vi "WIP.vi"() -> ()   [LabVIEW 2020]
uses:
  <vilib>/userdefined/High Color/IMAQdx.ctl
  Supporting Files/Sensor Station States.ctl
  Keyence CL-3000/Public/clusters/CL3IF_MEASUREMENT_DATA.ctl
  Keyence CL-3000/Public/clusters/CL3IF_OUTMEASUREMENT_DATA.ctl
  Keyence CL-3000/Public/enums/CL3IF_VALUE_INFO.ctl
  Keyence CL-3000/Public/enums/CL3IF_JUDGE_RESULT.ctl
  Keyence CL-3000/Public/clusters/CL3IF_ETHERNET_SETTING.ctl
  Keyence CL-3000/Keyence CL-3000.lvlib
  <vilib>/WebDAVClient/NI_WebDAV.lvlib
  <vilib>/vision/driver/NI_Vision_Acquisition_Software.lvlib
  <vilib>/WebDAVClient/Advanced/Multi Event/Asynchronous Get File.vi
panel:
  in  "Select Camera":T1
  in  "Enable Camera":bool
  in  "Visualise \nLaser":bool
  out "Numeric":i32
  out "Confocal\nSave Error":errorcluster
  in  "Visualise\nChromatic":bool
  in  "Log Laser Data":bool
  out "Laser Displacement Readings (cRIO) 2":dbl(graph)
  in  "Enable Laser":bool
  in  "Filename":string
  in  "Save Location (Folder)":path
  out "Chromatic Logged Data Points":u32
  in  "IP Address":u8[](array[numeric])=[192, 168, 1, 1]
  in  "Port":u32
  in  "timeout":u32=5000 caption="Timeout"
  in  "Comm Interface":enum8{"USB", "ETHERNET"}(ring)
  in  "Device ID":i32 min=0 max=2
  out "Confocal Data Index 2":u32
  in  "Log Chromatic Data":bool
  in  "Enable Chromatic":bool
  out "Confocal Data Index 1":u32
  in  "STOP":bool
  out "Camera Feed":T2(plugin-control)
  in  "Capture Image":bool
  out "Captured Image":T2(plugin-control)
  out "Measurement Data":T3(array[cluster])=[{"Out No"=1, "Value"=0, "valueInfo"=enum."VALID", "judgeResult"=0}, {"Out No"=2, "Value"=0, "valueInfo"=enum."VALID", "judgeResult"=0}, {"Out No"=3, "Value"=0, "valueInfo"=enum."VALID", "judgeResult"=0}, {"Out No"=4, "Value"=0, "valueInfo"=enum."VALID", "judgeResult"=0}, {"Out No"=5, "Value"=0, "valueInfo"=enum."VALID", "judgeResult"=0}, {"Out No"=6, "Value"=0, "valueInfo"=enum."VALID", "judgeResult"=0}, {"Out No"=7, "Value"=0, "valueInfo"=enum."VALID", "judgeResult"=0}, {"Out No"=8, "Value"=0, "valueInfo"=enum."VALID", "judgeResult"=0}] {"judgeResult" items=["HI"=1, "GO"=2, "LO"=4, "**"=5, "--"=0]}
  out "Chromatic Confocal Readings":dbl(graph)
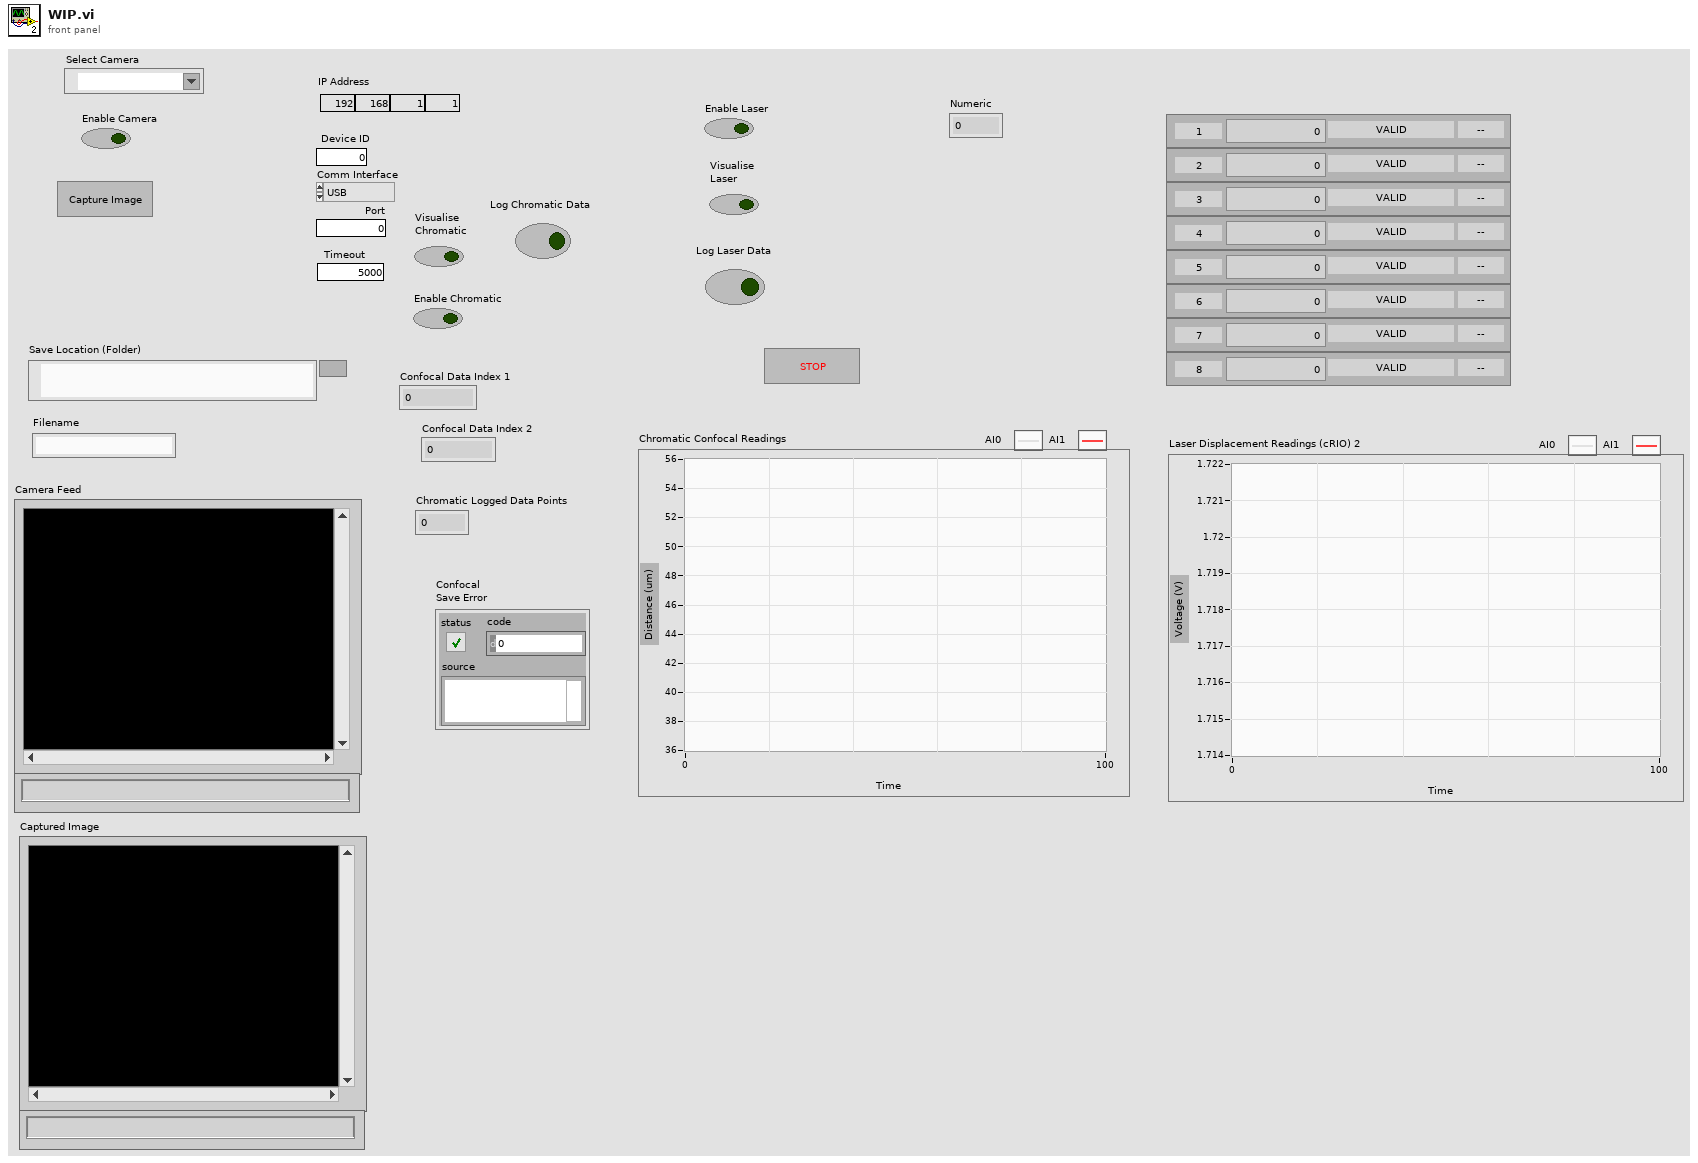
[diagram p1: front panel]
types:
  T1 = typedef "IMAQdx.ctl" = refnum<k21>
  T2 = typedef "IMAQ Image.ctl" = refnum<image>
  T3 = cluster{"Out No":i32, "Value":i32, "valueInfo":enum8{"VALID", "JUDGMENTSTANDBY", "INVALID", "OVERDISPRANGE_P", "OVERDISPRANGE_N"}, "judgeResult":u16}[]
  T4 = typedef "Keyence CL-3000.lvlib/CL3IF_MEASUREMENT_DATA.ctl" = cluster{"addInfo":cluster{"triggerCount":u32, "pulseCount":i32}, "outMeasurementData":T5[]}
  T5 = typedef "Keyence CL-3000.lvlib/CL3IF_OUTMEASUREMENT_DATA.ctl" = cluster{"measurementValue":i32, "valueInfo":T6, "judgeResult":T7}
  T6 = typedef "Keyence CL-3000.lvlib/CL3IF_VALUE_INFO.ctl" = enum8{"VALID", "JUDGMENTSTANDBY", "INVALID", "OVERDISPRANGE_P", "OVERDISPRANGE_N"}
  T7 = typedef "Keyence CL-3000.lvlib/CL3IF_JUDGE_RESULT.ctl" = u8
  T8 = typedef "Sensor Station States.ctl" = enum16{"Initialise", "Acquire", "Visualise", "Log", "Save", "Check Time", "Idle", "Close"}
  T9 = enum16{"open", "replace", "create", "open or create", "replace or create", "replace or create with confirmation"}
  T10 = typedef "NI_WebDAV.lvlib/Asynchronous Session Handle.ctl" = refnum<k1>
  T11 = typedef "Keyence CL-3000.lvlib/CL3IF_ETHERNET_SETTING.ctl" = cluster{"IP Address":cluster{"IP1":u8, "IP2":u8, "IP3":u8, "IP4":u8}, "portNo":u32}
  T12 = cluster{"IP Address":u8, "IP Address":u8, "IP Address":u8, "IP Address":u8}
  T13 = cluster{i32, "measurementValue":i32, "valueInfo":T6, "judgeResult":T7}
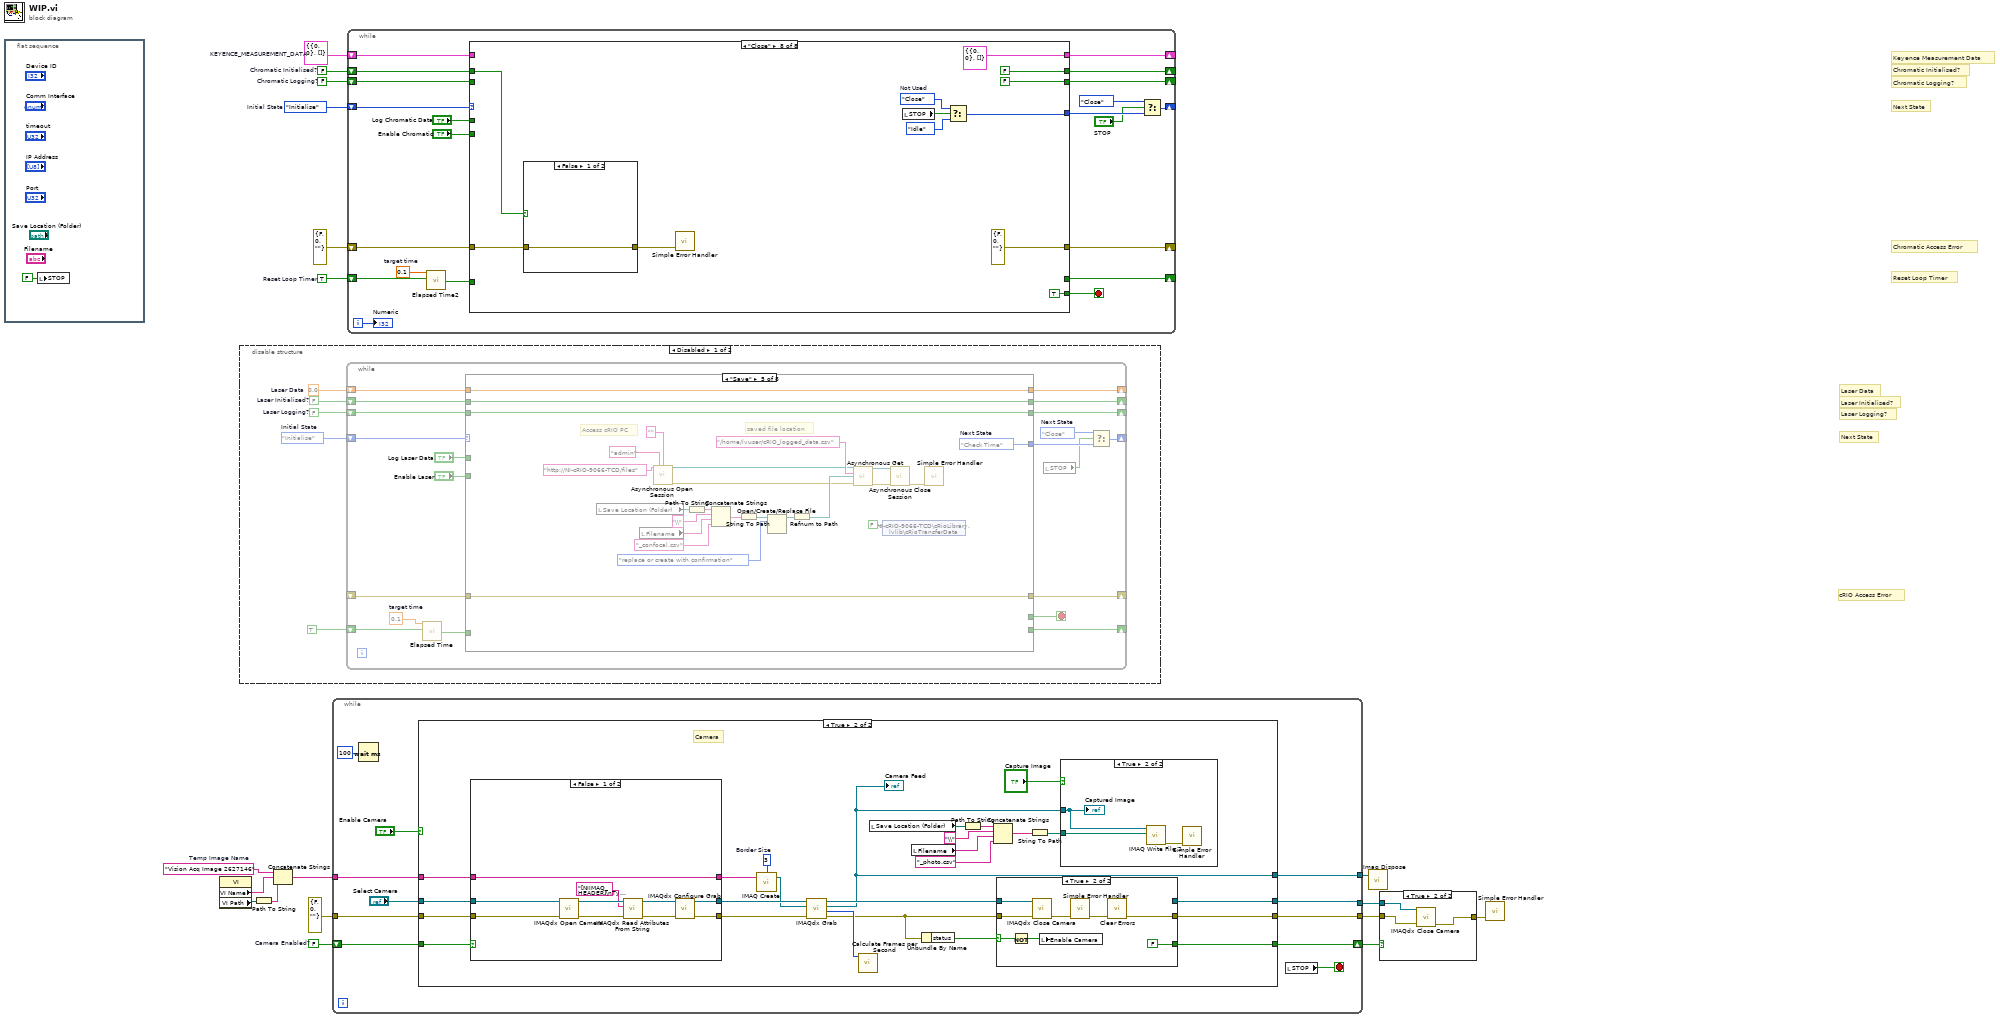
[diagram p0: block diagram]
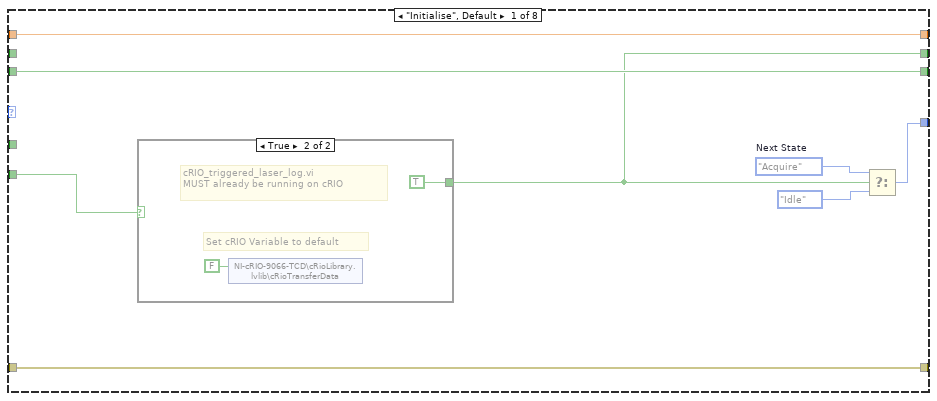
[diagram p3: hidden frame]
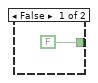
[diagram p4: hidden frame]
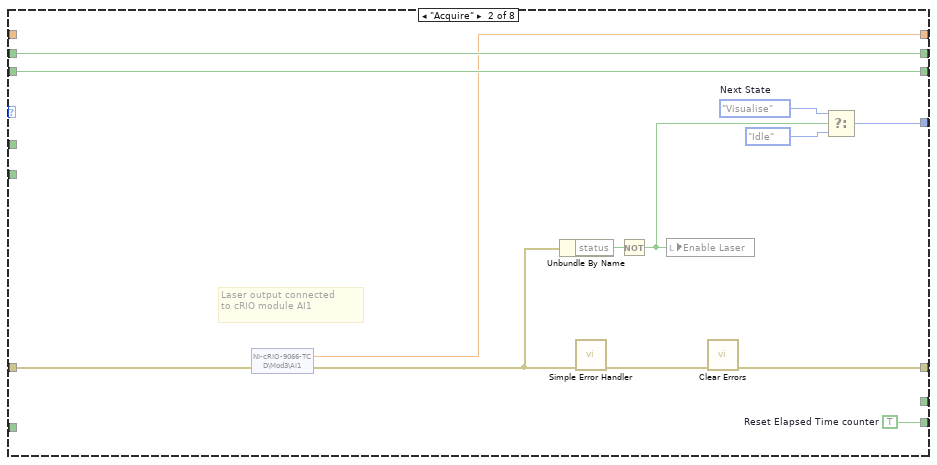
[diagram p5: hidden frame]
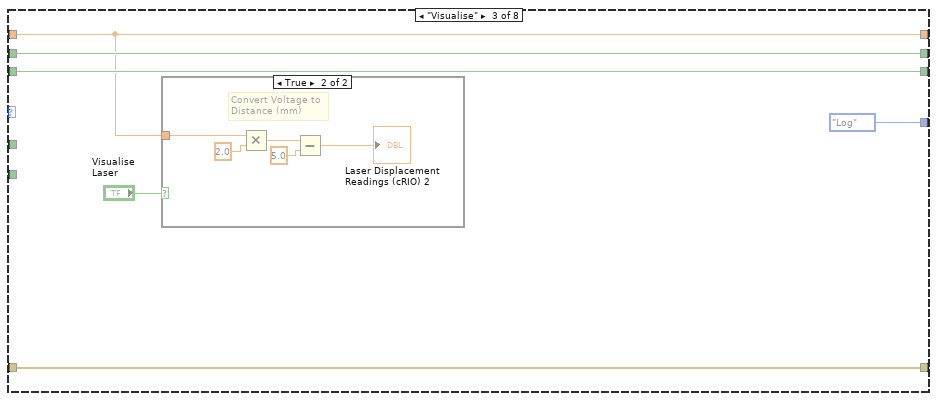
[diagram p6: hidden frame]
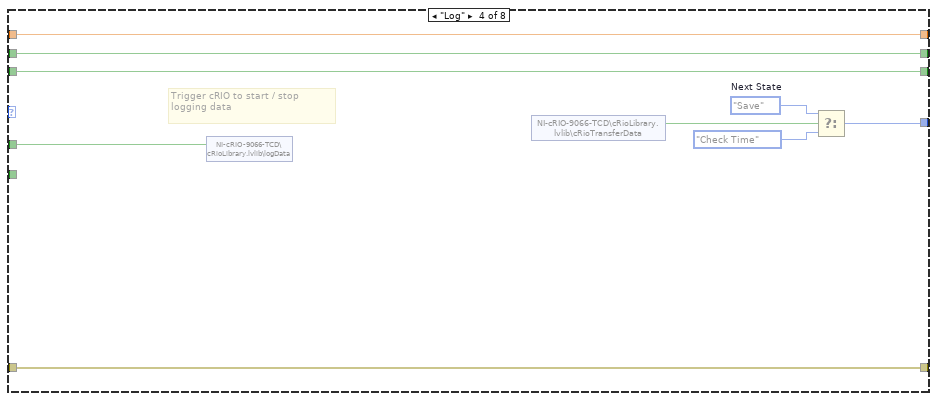
[diagram p8: hidden frame]
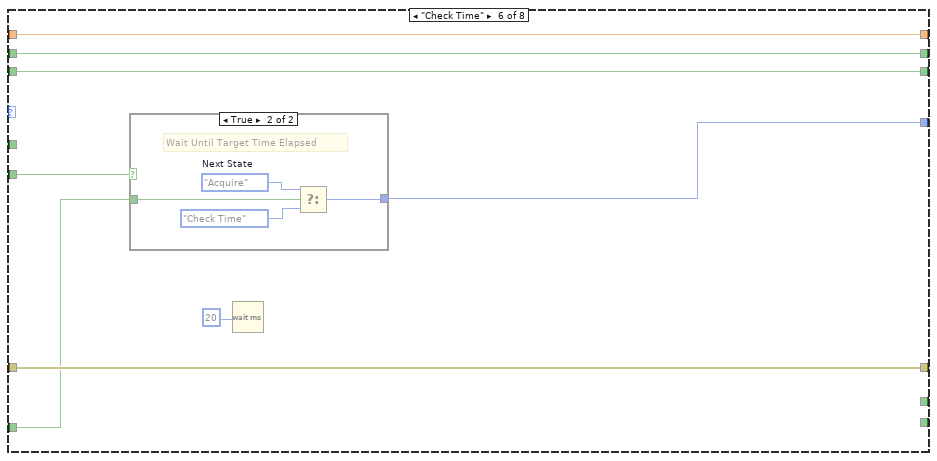
[diagram p9: hidden frame]
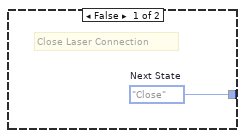
[diagram p10: hidden frame]
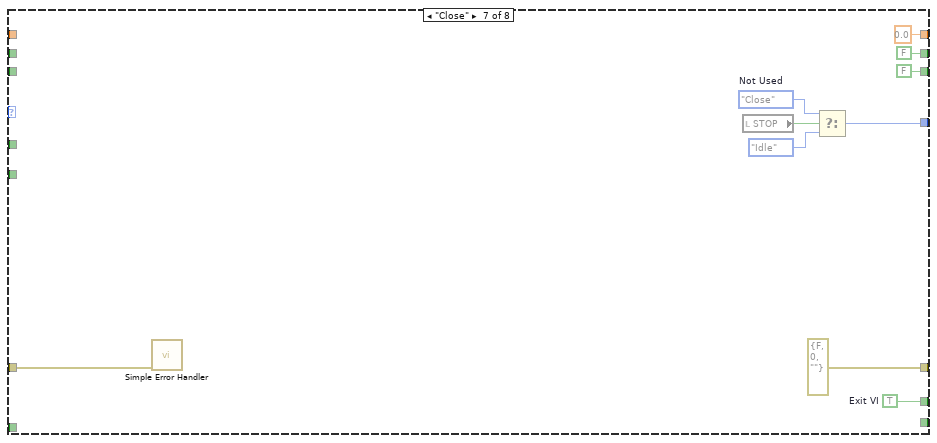
[diagram p11: hidden frame]
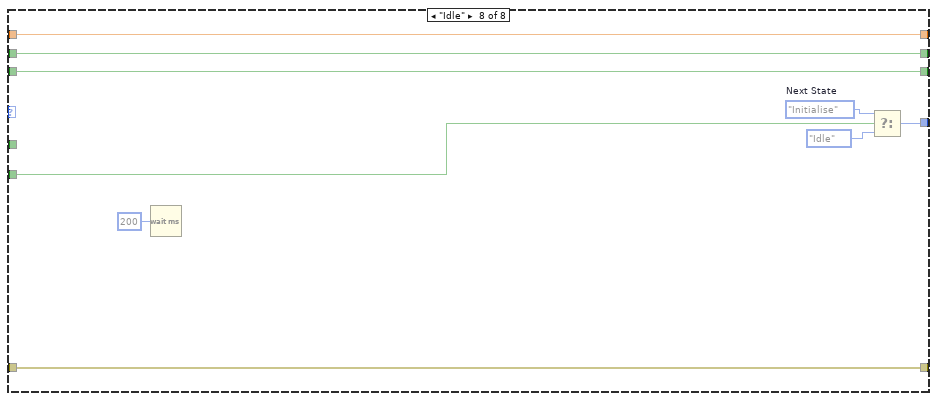
[diagram p12: hidden frame]
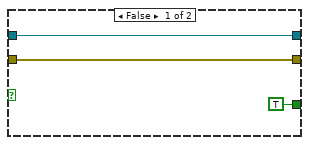
[diagram p16: hidden frame]
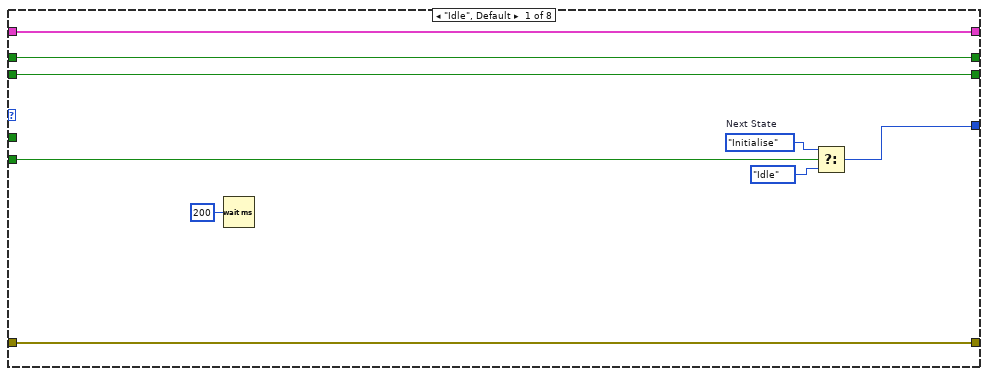
[diagram p18: hidden frame]
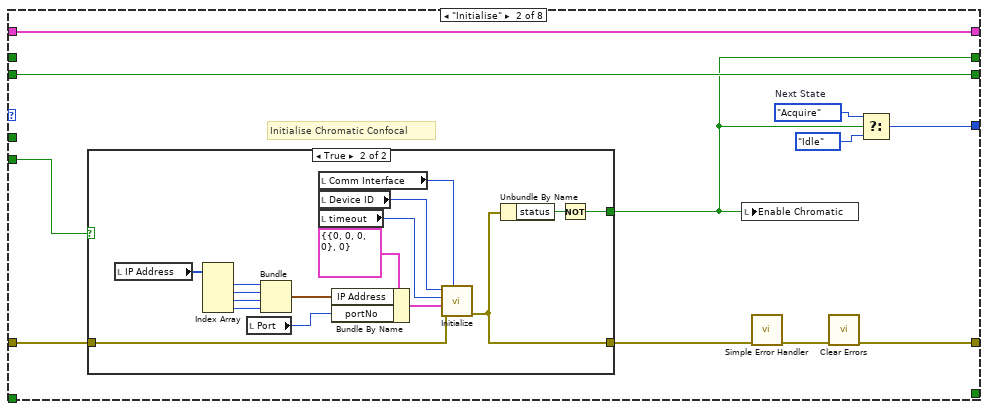
[diagram p19: hidden frame]
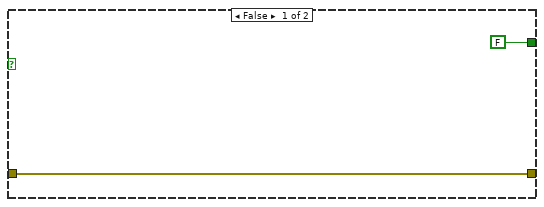
[diagram p20: hidden frame]
diagram:
  w7 = "Vision Acq Image 2627146"  # Temp Image Name
  w11 = FALSE  # Camera Enabled?
  w14 = FALSE  # Chromatic Initialised?
  w15 = FALSE  # Chromatic Logging?
  w16 = TRUE  # Reset Loop Timer
  w17 = T4 {"addInfo"={"triggerCount"=0, "pulseCount"=0}, "outMeasurementData"=[]}  # KEYENCE_MEASUREMENT_DATA
  w18 = Sensor_Station_States."Initialise"  # Initial State
  # "cRIO Access Error"
  # "Next State"
  # "Laser Logging?"
  # "Laser Initialised?"
  # "Laser Data"
  # "Reset Loop Timer"
  # "Chromatic Access Error"
  # "Next State"
  # "Keyence Measurement Data"
  # "Chromatic Logging?"
  # "Chromatic Initialised?"
  n1 = flat-sequence {
    frame #0 {
      n2 = local write "STOP"(FALSE ("STOP")) -> ()
    }
  }
  n3 = property class="VI"() -> ("VI Name"=w9:string, "VI Path"=w8:path)  [unwired: 2 in, 2 out]
  n4 = disable-structure shown="Disabled" {
    frame Disabled {
      w20 = 0.0  # Laser Data
      w21 = FALSE  # Laser Initialised?
      w24 = FALSE  # Laser Logging?
      w22 = Sensor_Station_States."Initialise"  # Initial State
      n5 = while {
        shift-right: [w31] -> _
        shift-left: w22 -> [w44]
        shift-right: [w40] -> _
        shift-left: TRUE -> [w42]
        shift-right: [w38] -> _
        shift-left: w24 -> [w39]
        shift-right: [w37] -> _
        shift-left: _ -> [w36]
        shift-right: [w35] -> _
        shift-left: w21 -> [w34]
        shift-right: [w27] -> _
        shift-left: w20 -> [w26]
        stop <- w30 stop-if-true
        w32 = Sensor_Station_States."Close"  # Next State
        w43 = 0.1  # target time
        n6 = call "Elapsed Time"("Time Target (s)"=w43, "Reset"=w42) -> ("Time has Elapsed"=w41:bool)  [unwired: 10 in, 7 out]
        n7 = case shown="\"Save\"" w44 {
          tunnel: w36 -> [w46 w67 w73 w83 w113 w118 w127 w140]
          tunnel: [w51 w57 Sensor_Station_States."Log" ("Next State") w86 w112 w115 w129 w142] -> w33
          tunnel: w41 -> [_ _ _ _ _ w116 _ _]
          tunnel: [_ w68 _ _ _ _ _ _] -> w40
          tunnel: w39 -> [w50 w65 w72 w81 w109 w120 _ w138]
          tunnel: [w50 w65 w72 w81 w109 w120 FALSE ("Chromatic Logging?") w138] -> w38
          tunnel: [w46 w62 w73 w83 w113 w118 errorcluster {"status"=FALSE, "code"=0, "source"=""} ("error constant") w140] -> w37
          tunnel: [w48 w66 w74 w88 w110 w119 FALSE w139] -> w35
          tunnel: w34 -> [_ w66 w74 w88 w110 w119 _ w139]
          tunnel: [_ _ _ _ _ _ w136 _] -> w30
          tunnel: "Enable Laser" -> [w49 _ _ _ _ w117 _ w143]
          tunnel: [w45 w64 w69 w82 w111 w114 0.0 w137] -> w27
          tunnel: w26 -> [w45 _ w69 w82 w111 w114 _ w137]
          tunnel: "Log Laser Data" -> [_ _ _ w84 _ _ _ _]
          frame "Initialise", Default {
            w47 = Sensor_Station_States."Acquire"  # Next State
            n8 = case shown="True" w49 {
              tunnel: [FALSE TRUE] -> w48
              frame False {
              }
              frame True {
                # "cRIO_triggered_laser_log.vi \nMUST already be running on cRIO"
                # "Set cRIO Variable to default"
                n9 = shared-variable "NI-cRIO-9066-TCD\\cRioLibrary.lvlib\\cRioTransferData"(FALSE ("cRioTransferData")) -> ()  [unwired: 1 in, 1 out]
              }
            }
            n10 = Select(t=w47, s=w48, f=Sensor_Station_States."Idle" ("Next State")) -> (s? t:f=w51:T8)
          }
          frame "Acquire" {
            w68 = TRUE  # Reset Elapsed Time counter
            w58 = Sensor_Station_States."Visualise"  # Next State
            # "Laser output connected \nto cRIO module AI1"
            n11 = shared-variable "NI-cRIO-9066-TCD\\Mod3\\AI1"(error in=w67) -> (w64:dbl, error out=w60:errorcluster)
            n12 = Unbundle By Name(w60) -> ("status"=w61:bool)
            n13 = call <vilib>:"Simple Error Handler.vi"("error in (no error)"=w60) -> ("error out"=w63:errorcluster)  [unwired: 4 in, 4 out]
            n14 = Not(x=w61) -> (.not. x?=w59:bool)
            n15 = local write "Enable Laser"(w59) -> ()
            n16 = call <vilib>:"Clear Errors.vi"("error in (no error)"=w63) -> ("error out"=w62:errorcluster)  [unwired: 5 in, 1 out]
            n17 = Select(t=w58, s=w59, f=Sensor_Station_States."Idle" ("Next State")) -> (s? t:f=w57:T8)
          }
          frame "Visualise" {
            n18 = case shown="True" "Visualise \nLaser" {
              tunnel: w69 -> [_ w75]
              frame False {
                # "Do nothing"
              }
              frame True {
                # "Convert Voltage to Distance (mm)"
                n19 = Multiply(x=w75, y=2.0) -> (x*y=w78:dbl)
                n20 = Subtract(x=w78, y=5.0) -> (x-y=→"Laser Displacement Readings (cRIO) 2":dbl)
              }
            }
          }
          frame "Log" {
            w87 = Sensor_Station_States."Save"  # Next State
            # "Trigger cRIO to start / stop \nlogging data"
            n21 = shared-variable "NI-cRIO-9066-TCD\\cRioLibrary.lvlib\\logData"(w84) -> ()  [unwired: 1 in, 1 out]
            n22 = shared-variable "NI-cRIO-9066-TCD\\cRioLibrary.lvlib\\cRioTransferData"() -> (w80:bool)  [unwired: 1 in, 1 out]
            n23 = Select(t=w87, s=w80, f=Sensor_Station_States."Check Time" ("Next State")) -> (s? t:f=w86:T8)
          }
          frame "Save" {
            w112 = Sensor_Station_States."Check Time"  # Next State
            # "Access cRIO PC"
            # "saved file location"
            n24 = local read "Save Location (Folder)"() -> (w106:path)
            n25 = local read "Filename"() -> (w103:string)
            n26 = call <vilib>:"Asynchronous Open Session.vi"("host uri prefix"="http://NI-cRIO-9066-TCD/files", "username"="admin", "password"="") -> ("session handle out"=w93:T10, "error out"=w92:errorcluster)  [unwired: 10 in, 1 out]
            n27 = Path To String(path=w106) -> (string=w105:string)
            n28 = Concatenate Strings(w105, "\\" ("string"), w103, "_confocal.csv" ("string")) -> (w101:string)
            n29 = String To Path(string=w101) -> (path=w100:path)
            n30 = Open/Create/Replace File(file path (use dialog)=w100, operation (0:open)=T9."replace or create with confirmation") -> (refnum out=w98:refnum<file>)  [unwired: 4 in, 2 out]
            n31 = Refnum to Path(1:w98) -> (0:w97:path)
            n32 = call-poly <vilib>:"Asynchronous Get.vi"("session handle"=w93, "relative uri"="/home/lvuser/cRIO_logged_data.csv", "local file path"=w97, "error in (no error)"=w92) -> ("session handle out"=w90:T10, "error out"=w89:errorcluster)  [unwired: 8 in, 2 out]
            n33 = shared-variable "NI-cRIO-9066-TCD\\cRioLibrary.lvlib\\cRioTransferData"(FALSE ("cRioTransferData")) -> ()  [unwired: 1 in, 1 out]
            n34 = call <vilib>:"Asynchronous Close Session.vi"("session handle"=w90, "error in (no error)"=w89) -> ("error out"=w91:errorcluster)  [unwired: 13 in]
            n35 = call <vilib>:"Simple Error Handler.vi"("error in (no error)"=w91) -> ()  [unwired: 4 in, 5 out]
          }
          frame "Check Time" {
            n36 = case shown="True" w117 {
              tunnel: w116 -> [_ w124]
              tunnel: [w122 w123] -> w115
              frame False {
                w122 = Sensor_Station_States."Close"  # Next State
                # "Close Laser Connection"
              }
              frame True {
                w125 = Sensor_Station_States."Acquire"  # Next State
                # "Wait Until Target Time Elapsed"
                n37 = Select(t=w125, s=w124, f=Sensor_Station_States."Check Time" ("Next State")) -> (s? t:f=w123:T8)
              }
            }
            n38 = Wait (ms)(milliseconds to wait=u32 20) -> ()  [unwired: 1 out]
          }
          frame "Close" {
            w131 = Sensor_Station_States."Close"  # Not Used
            w136 = TRUE  # Exit VI
            n39 = call <vilib>:"Simple Error Handler.vi"("error in (no error)"=w127) -> ()  [unwired: 4 in, 5 out]
            n40 = local read "STOP"() -> (w130:bool)
            n41 = Select(t=w131, s=w130, f=Sensor_Station_States."Idle" ("Next State")) -> (s? t:f=w129:T8)
          }
          frame "Idle" {
            w145 = Sensor_Station_States."Initialise"  # Next State
            n42 = Wait (ms)(milliseconds to wait=u32 200) -> ()  [unwired: 1 out]
            n43 = Select(t=w145, s=w143, f=Sensor_Station_States."Idle" ("Next State")) -> (s? t:f=w142:T8)
          }
        }
        n44 = local read "STOP"() -> (w29:bool)
        n45 = Select(t=w32, s=w29, f=w33) -> (s? t:f=w31:T8)
      }
    }
    frame Enabled {
    }
  }
  n46 = Path To String(path=w8) -> (string=w10:string)
  n47 = Concatenate Strings(w7, w9, w10) -> (w6:string)
  n48 = while {
    tunnel: [w156] -> w12
    tunnel: [w155] -> w3
    shift-right: [w147] -> w1
    shift-left: w11 -> [w151]
    tunnel: errorcluster {"status"=FALSE, "code"=0, "source"=""} ("error in") -> [w149]
    tunnel: w6 -> [w150]
    tunnel: [w146] -> w4
    stop <- w152 stop-if-true
    n49 = Wait (ms)(milliseconds to wait=u32 100) -> ()  [unwired: 1 out]
    n50 = case shown="True" "Enable Camera" {
      tunnel: [w158 w183] -> w155
      tunnel: [_ w170] -> w156
      tunnel: w151 -> [w157 w169]
      tunnel: w150 -> [_ w164]
      tunnel: w149 -> [w158 w168]
      tunnel: "Select Camera" -> [w159 w163]
      tunnel: [w157 w161] -> w147
      tunnel: [w159 w160] -> w146
      frame False {
      }
      frame True {
        w167 = 3  # Border Size
        # "Camera"
        n51 = case shown="False" w169 {
          tunnel: [w194 w196] -> w177
          tunnel: [w193 w195] -> w176
          tunnel: w168 -> [w187 w195]
          tunnel: [w186 w197] -> w165
          tunnel: w164 -> [w186 w197]
          tunnel: w163 -> [w185 w196]
          frame False {
            n52 = call <vilib>:"IMAQdx Open Camera.vi"("error in"=w187, "Session In"=w185) -> ("error out"=w191:errorcluster, "Session Out"=w192:T1)  [unwired: 1 in, 7 out]
            n53 = call <vilib>:"IMAQdx Read Attributes From String.vi"("error in"=w191, "Attributes String In"="[NIIMAQ_HEADER]\nType = 2\nVersion = 8\n\n[CAMERA_DATA]\nAcquisitionAttributes::Bayer::Algorithm = \"Bilinear\"\nAcquisitionAttributes::Bayer::GainB = \"1\"\nAcquisitionAttributes::Bayer::GainG = \"1\"\nAcquisitionAttributes::Bayer::GainR = \"1\"\nAcquisitionAttributes::Bayer::Pattern = \"Use hardware value\"\nAcquisitionAttributes::BitsPerPixel = \"Use hardware value\"\nAcquisitionAttributes::HardwareMaximumQueuedBufferCount = \"1000\"\nAcquisitionAttributes::HardwareRequeueBufferListThreshold = \"50\"\nAcquisitionAttributes::IgnoreFirstFrame = \"false\"\nAcquisitionAttributes::ImageDecoderCopyMode = \"Auto\"\nAcquisitionAttributes::OutputImageType = \"Auto\"\nAcquisitionAttributes::OverwriteMode = \"Get Newest\"\nAcquisitionAttributes::PixelSignedness = \"Use hardware value\"\nAcquisitionAttributes::ReceiveTimestampMode = \"None\"\nAcquisitionAttributes::ShiftPixelBits = \"false\"\nAcquisitionAttributes::SwapPixelBytes = \"false\"\nAcquisitionAttributes::Timeout = \"5000\"\nAcquisitionAttributes::VerticalMirror = \"false\"\nAcquisitionAttributes::VideoMode = \"640x480 YUY2 30.00fps\"\nCameraAttributes::BacklightCompensation::Mode = \"Manual\"\nCameraAttributes::BacklightCompensation::Value = \"true\"\nCameraAttributes::Brightness::Mode = \"Manual\"\nCameraAttributes::Brightness::Value = \"0\"\nCameraAttributes::Contrast::Mode = \"Manual\"\nCameraAttributes::Contrast::Value = \"0.179999999999999993\"\nCameraAttributes::Exposure::Mode = \"Auto\"\nCameraAttributes::Gain::Mode = \"Manual\"\nCameraAttributes::Gain::Value = \"1\"\nCameraAttributes::Gamma::Mode = \"Manual\"\nCameraAttributes::Gamma::Value = \"1.5\"\nCameraAttributes::Hue::Mode = \"Manual\"\nCameraAttributes::Hue::Value = \"0\"\nCameraAttributes::Saturation::Mode = \"Manual\"\nCameraAttributes::Saturation::Value = \"8\"\nCameraAttributes::Sharpness::Mode = \"Manual\"\nCameraAttributes::Sharpness::Value = \"3\"\nCameraAttributes::WhiteBalance::Mode = \"Auto\"\n" ("Attributes"), "Session In"=w192) -> ("error out"=w189:errorcluster, "Session Out"=w190:T1)  [unwired: 7 out]
            n54 = call <vilib>:"IMAQdx Configure Grab.vi"("error in"=w189, "Session In"=w190) -> ("error out"=w193:errorcluster, "Session Out"=w194:T1)  [unwired: 1 in, 7 out]
          }
          frame True {
            # "Camera Initialised"
          }
        }
        n55 = call "IMAQ Create"("Border Size"=w167, "Image Name"=w165) -> ("New Image"=w166:T2)  [unwired: 2 in, 2 out]
        n56 = call <vilib>:"IMAQdx Grab.vi"("error in"=w176, "Image In"=w166, "Session In"=w177) -> ("error out"=w178:errorcluster, "Buffer Number Out"=w179:u32, "Image Out"=w170:T2, "Session Out"=w180:T1)  [unwired: 1 in, 4 out]
        "Camera Feed" <- w170
        n57 = call <vilib>:"Calculate Frames per Second.vi"("Buffer Number"=w179) -> ()  [unwired: 2 in, 9 out]
        n58 = local read "Save Location (Folder)"() -> (w175:path)
        n59 = local read "Filename"() -> (w172:string)
        n60 = Unbundle By Name(w178) -> ("status"=w162:bool)
        n61 = Path To String(path=w175) -> (string=w174:string)
        n62 = Concatenate Strings(w174, "\\" ("string"), w172, "_photo.csv" ("string")) -> (w182:string)
        n63 = case "Case Structure_template1" shown="True" w162 {
          selector: w162 -> [_ w203]
          tunnel: [w200 w204] -> w183
          tunnel: w178 -> [w200 w208]
          tunnel: w180 -> [w198 w206]
          tunnel: [TRUE FALSE] -> w161
          tunnel: [w198 _] -> w160
          frame False {
          }
          frame True {
            n64 = Not(x=w203) -> (.not. x?=w202:bool)
            n65 = call <vilib>:"IMAQdx Close Camera.vi"("error in"=w208, "Session In"=w206) -> ("error out"=w207:errorcluster)  [unwired: 9 out]
            n66 = local write "Enable Camera"(w202) -> ()
            n67 = call <vilib>:"Simple Error Handler.vi"("error in (no error)"=w207) -> ("error out"=w205:errorcluster)  [unwired: 4 in, 4 out]
            n68 = call <vilib>:"Clear Errors.vi"("error in (no error)"=w205) -> ("error out"=w204:errorcluster)  [unwired: 5 in, 1 out]
          }
        }
        n69 = String To Path(string=w182) -> (path=w181:path)
        n70 = case shown="True" "Capture Image" {
          tunnel: w170 -> [_ w211]
          tunnel: w181 -> [_ w210]
          frame False {
          }
          frame True {
            n71 = call-poly "IMAQ Write File 2"("File Path"=w210, "Image"=w211) -> ("error out"=w209:errorcluster)  [unwired: 8 in, 1 out]
            n72 = call <vilib>:"Simple Error Handler.vi"("error in (no error)"=w209) -> ()  [unwired: 4 in, 5 out]
            "Captured Image" <- w211
          }
        }
      }
    }
    n73 = local read "STOP"() -> (w152:bool)
  }
  n74 = while {
    shift-right: [w217] -> _
    shift-left: w18 -> [w232]
    shift-right: [w230] -> _
    shift-left: w17 -> [w231]
    shift-right: [w226] -> _
    shift-left: w16 -> [w228]
    shift-right: [w224] -> _
    shift-left: w15 -> [w225]
    shift-right: [w223] -> _
    shift-left: errorcluster {"status"=FALSE, "code"=0, "source"=""} ("error constant") -> [w222]
    shift-right: [w221] -> _
    shift-left: w14 -> [w220]
    i -> [w212]
    stop <- w216 stop-if-true
    w229 = 0.1  # target time
    n75 = call "Elapsed Time2"("Time Target (s)"=w229, "Reset"=w228) -> ("Time has Elapsed"=w227:bool)  [unwired: 10 in, 7 out]
    n76 = case shown="\"Close\"" w232 {
      tunnel: w231 -> [w240 w252 _ w279 w308 w352 w377 _]
      tunnel: w222 -> [w234 w248 w276 w283 w311 w342 w380 w400]
      tunnel: [w240 w252 w272 w279 w308 w352 w377 T4 {"addInfo"={"triggerCount"=0, "pulseCount"=0}, "outMeasurementData"=[]} ("KEYENCE_MEASUREMENT_DATA")] -> w230
      tunnel: [w237 w250 w275 Sensor_Station_States."Log" ("Next State") w304 w341 w378 w393] -> w219
      tunnel: w227 -> [_ _ _ _ _ _ w379 _]
      tunnel: [_ _ w278 _ _ _ _ _] -> w226
      tunnel: w225 -> [w233 w249 w277 w282 w312 w339 w382 _]
      tunnel: [w233 w249 w277 w282 w310 w339 w382 FALSE ("Chromatic Logging?")] -> w224
      tunnel: [w234 w244 w273 w283 w301 w342 w380 errorcluster {"status"=FALSE, "code"=0, "source"=""} ("error constant")] -> w223
      tunnel: [w241 w243 w271 w284 w309 w340 w381 FALSE] -> w221
      tunnel: w220 -> [w241 _ w271 w284 w309 w340 w381 w392]
      tunnel: [_ _ _ _ _ _ _ TRUE ("Exit VI")] -> w216
      tunnel: "Enable Chromatic" -> [w236 w246 _ _ _ _ w376 _]
      tunnel: "Log Chromatic Data" -> [_ _ _ _ w303 _ _ _]
      frame "Idle", Default {
        w239 = Sensor_Station_States."Initialise"  # Next State
        n77 = Wait (ms)(milliseconds to wait=u32 200) -> ()  [unwired: 1 out]
        n78 = Select(t=w239, s=w236, f=Sensor_Station_States."Idle" ("Next State")) -> (s? t:f=w237:T8)
      }
      frame "Initialise" {
        w251 = Sensor_Station_States."Acquire"  # Next State
        # "Initialise Chromatic Confocal"
        n79 = case shown="True" w246 {
          tunnel: [w253 w257] -> w245
          tunnel: [FALSE w256] -> w243
          tunnel: w248 -> [w253 w258]
          frame False {
          }
          frame True {
            n80 = local read "IP Address"() -> (w260:u8[])
            n81 = Index Array(array=w260) -> (element #1=w265:u8, element #2=w266:u8, element #3=w267:u8, element #4=w268:u8)  [unwired: 4 in]
            n82 = local read "Port"() -> (w259:u32)
            n83 = Bundle("IP Address"=w265, "IP Address"=w266, "IP Address"=w267, "IP Address"=w268) -> (w269:T12)  [unwired: 1 in]
            n84 = local read "Comm Interface"() -> (w262:enum8{"USB", "ETHERNET"})
            n85 = local read "Device ID"() -> (w263:i32)
            n86 = local read "timeout"() -> (w261:u32)
            n87 = Bundle By Name(cluster=T11 {"IP Address"={"IP1"=0, "IP2"=0, "IP3"=0, "IP4"=0}, "portNo"=0} ("ethernetSetting"), "IP Address"=w269, "portNo"=w259) -> (w270:T11)
            n88 = call "Initialize.vi"("Comm Interface"=w262, "error in (no error)"=w258, "ethernetSetting"=w270, "timeout"=w261, "deviceId"=w263) -> ("error out"=w257:errorcluster)  [unwired: 6 in]
            n89 = Unbundle By Name(w257) -> ("status"=w255:bool)
            n90 = Not(x=w255) -> (.not. x?=w256:bool)
          }
        }
        n91 = local write "Enable Chromatic"(w243) -> ()
        n92 = call <vilib>:"Simple Error Handler.vi"("error in (no error)"=w245) -> ("error out"=w242:errorcluster)  [unwired: 4 in, 4 out]
        n93 = call <vilib>:"Clear Errors.vi"("error in (no error)"=w242) -> ("error out"=w244:errorcluster)  [unwired: 5 in, 1 out]
        n94 = Select(t=w251, s=w243, f=Sensor_Station_States."Idle" ("Next State")) -> (s? t:f=w250:T8)
      }
      frame "Acquire" {
        w275 = Sensor_Station_States."Visualise"  # Next State
        w278 = TRUE  # Reset Elapsed Time counter
        n95 = local read "Device ID"() -> (w274:i32)
        n96 = call "CL3IF_GetMeasurementData.vi"("error in"=w276, "deviceId"=w274) -> ("error out"=w273:errorcluster, "MEASUREMENT_DATA"=w272:T4)  [unwired: 8 in]
      }
      frame "Visualise" {
        n97 = case shown="True" "Visualise\nChromatic" {
          tunnel: w279 -> [_ w286]
          frame False {
            # "Do Nothing"
          }
          frame True {
            n98 = Unbundle By Name(w286) -> ("outMeasurementData"=w292:T5[])
            n99 = Index Array(array=w292, index=0) -> (element=w291:T5)
            n100 = for {
              tunnel: w292 -> [w300] mode=indexing
              tunnel: [w299] -> w293 mode=indexing
              i -> [w298]
              n101 = Unbundle By Name(w300) -> ("measurementValue"=w294:i32, "valueInfo"=w296:T6, "judgeResult"=w295:T7)
              n102 = Increment(x=w298) -> (x+1=w297:i32)
              n103 = Bundle(w297, "measurementValue"=w294, "valueInfo"=w296, "judgeResult"=w295) -> (w299:T13)  [unwired: 1 in]
            }
            "Measurement Data" <- w293
            n104 = Unbundle By Name(w291) -> ("measurementValue"=w290:i32)
            n105 = To Double Precision Float(number=w290) -> (double precision float=w285:dbl)
            n106 = Divide(x=w285, y=1000.0) -> (x/y=→"Chromatic Confocal Readings":dbl)
          }
        }
      }
      frame "Log" {
        w306 = Sensor_Station_States."Save"  # Next State
        n107 = local read "Device ID"() -> (w302:i32)
        n108 = case shown="True" w303 {
          tunnel: w312 -> [w317 w331]
          tunnel: w311 -> [w318 w330]
          tunnel: [w316 w329] -> w301
          tunnel: [FALSE TRUE] -> w310
          tunnel: [w314 FALSE ("conSaveData")] -> w307
          tunnel: w302 -> [w313 w326]
          frame False {
            n109 = case shown="True" w317 {
              tunnel: w318 -> [w320 w324]
              tunnel: [w320 w322] -> w316
              tunnel: [FALSE ("conSaveData") TRUE ("conSaveData")] -> w314
              tunnel: w313 -> [_ w321]
              frame False {
                # "Not Logging\nDo nothing"
              }
              frame True {
                # "Move to Save State"
                # "Stop Logging & Record Data Index"
                n110 = call "CL3IF_GetTrendIndex.vi"("error in"=w324, "deviceId"=w321) -> ("error out"=w322:errorcluster, "index"=→"Confocal Data Index 2":u32)  [unwired: 8 in]
              }
            }
          }
          frame True {
            n111 = case shown="False" w331 {
              tunnel: w330 -> [w334 w336]
              tunnel: [w333 w336] -> w329
              tunnel: w326 -> [w332 _]
              frame False {
                # "Start Logging"
                n112 = call "CL3IF_GetTrendIndex.vi"("error in"=w334, "deviceId"=w332) -> ("error out"=w333:errorcluster, "index"=→"Confocal Data Index 1":u32)  [unwired: 8 in]
              }
              frame True {
                # "Currently Logging\nDo nothing"
              }
            }
          }
        }
        n113 = Select(t=w306, s=w307, f=Sensor_Station_States."Check Time" ("Next State")) -> (s? t:f=w304:T8)
      }
      frame "Save" {
        w341 = Sensor_Station_States."Check Time"  # Next State
        n114 = local read "Save Location (Folder)"() -> (w349:path)
        n115 = local read "Confocal Data Index 1"() -> (w351:u32)
        n116 = local read "Confocal Data Index 2"() -> (w350:u32)
        n117 = local read "Filename"() -> (w346:string)
        n118 = local read "Device ID"() -> (w337:i32)
        n119 = Path To String(path=w349) -> (string=w348:string)
        n120 = Concatenate Strings(w348, "\\" ("string"), w346, "_confocal.csv" ("string")) -> (w344:string)
        n121 = Subtract(x=w350, y=w351) -> (x-y=w359:u32)
        "Chromatic Logged Data Points" <- w359
        n122 = String To Path(string=w344) -> (path=w343:path)
        n123 = call "CL3IF_GetTrendData.vi"("requestDataCount"=w359, "index"=w351, "deviceId"=w337) -> ("measurementData"=w358:T4[])  [unwired: 4 in, 4 out]
        n124 = Open/Create/Replace File(file path (use dialog)=w343, operation (0:open)=T9."replace or create with confirmation") -> (refnum out=w357:refnum<file>, error out=w354:errorcluster)  [unwired: 4 in, 1 out]
        n125 = for {
          tunnel: w358 -> [w375] mode=indexing
          tunnel: w357 -> [w364]
          tunnel: [w362] -> w356
          tunnel: w354 -> [w361]
          tunnel: [w360] -> w353
          n126 = Unbundle By Name(w375) -> ("outMeasurementData"=w373:T5[])
          n127 = Index Array(array=w373, index=0) -> (element=w372:T5)
          n128 = Unbundle By Name(w372) -> ("measurementValue"=w369:i32)
          n129 = To Double Precision Float(number=w369) -> (double precision float=w370:dbl)
          n130 = Divide(x=w370, y=1000.0) -> (x/y=w368:dbl)
          n131 = Format Into String(format string="%.6f%s", error in=w361, w368, "\r\n") -> (resulting string=w365:string, error out=w363:errorcluster)  [unwired: 1 in]
          n132 = Write to Text File(file (use dialog)=w364, text=w365, error in=w363) -> (refnum out=w362:refnum<file>, error out=w360:errorcluster)  [unwired: 1 in, 1 out]
        }
        n133 = Close File(refnum=w356, error in=w353) -> (error out=→"Confocal\nSave Error":errorcluster)  [unwired: 1 out]
      }
      frame "Check Time" {
        n134 = case shown="True" w376 {
          tunnel: w379 -> [_ w386]
          tunnel: [w384 w385] -> w378
          frame False {
            w384 = Sensor_Station_States."Close"  # Next State
            # "Close Chromatic Connection"
          }
          frame True {
            w387 = Sensor_Station_States."Acquire"  # Next State
            # "Wait Until Target Time Elapsed"
            n135 = Select(t=w387, s=w386, f=Sensor_Station_States."Check Time" ("Next State")) -> (s? t:f=w385:T8)
          }
        }
        n136 = Wait (ms)(milliseconds to wait=u32 50) -> ()  [unwired: 1 out]
      }
      frame "Close" {
        w395 = Sensor_Station_States."Close"  # Not Used
        n137 = case shown="False" w392 {
          tunnel: w400 -> [w401 w404]
          tunnel: [w401 w402] -> w391
          frame False {
          }
          frame True {
            n138 = local read "Device ID"() -> (w403:i32)
            n139 = call "Close.vi"("error in (no error)"=w404, "deviceId"=w403) -> ("error out"=w402:errorcluster)  [unwired: 9 in]
          }
        }
        n140 = call <vilib>:"Simple Error Handler.vi"("error in (no error)"=w391) -> ()  [unwired: 4 in, 5 out]
        n141 = local read "STOP"() -> (w396:bool)
        n142 = Select(t=w395, s=w396, f=Sensor_Station_States."Idle" ("Next State")) -> (s? t:f=w393:T8)
      }
    }
    n143 = Select(t=Sensor_Station_States."Close" ("Next State"), s="STOP", f=w219) -> (s? t:f=w217:T8)
    "Numeric" <- w212
  }
  n144 = call "Imaq Dispose"("Image"=w12) -> ()  [unwired: 5 in, 1 out]
  n145 = case shown="True" w1 {
    tunnel: w4 -> [_ w408]
    tunnel: w3 -> [w405 w406]
    tunnel: [w405 w407] -> w2
    frame False {
    }
    frame True {
      n146 = call <vilib>:"IMAQdx Close Camera.vi"("error in"=w406, "Session In"=w408) -> ("error out"=w407:errorcluster)  [unwired: 9 out]
    }
  }
  n147 = call <vilib>:"Simple Error Handler.vi"("error in (no error)"=w2) -> ()  [unwired: 4 in, 5 out]
